vi "Administrator Console.vi"(8 "error in (no error)":errorcluster, 11 "Message Queues":T1) -> (0 "error out":errorcluster)   [LabVIEW 2024]
doc: "This VI is a user interface VI and is used to configure the server."
uses:
  Shared/Message Queue/Server Message Queues.ctl
  Shared/Message Queue/Message Cluster.ctl
  Controls/Server/Administrator Console - Data.ctl
  Shared/User Event - Stop.lvlib
  Shared/Message Queue.lvlib
panel:
  in  "Close":bool
  in  "Subsystems and I/O Points":string(tree)="..."
  in  "Configure Data Archiving":bool
  in  "Configure System":bool
  # "The Subsystem and I/O Points box lists every subsystem in the server and its I/O points. You can expand a subsystem to view its I/O points . Use the configuration buttons to modify the server."
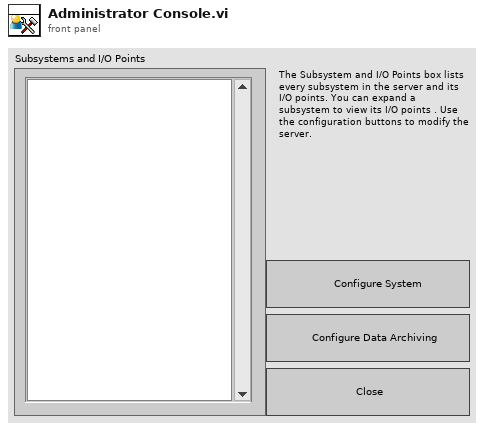
[diagram p1: front panel]
types:
  T1 = typedef "Message Queue.lvlib/Server Message Queues.ctl" = cluster{"UI":refnum<queue>, "Archive":refnum<queue>, "Shared Variable Management":refnum<queue>, "Administrator Console":refnum<queue>}
  T2 = typedef "Administrator Console - Data.ctl" = cluster{"Administrator Console Exit Handler":refnum<user-event>, "Server Message Queues":T1, "Subsystems Tree Control":refnum<vi>}
  T3 = typedef "Subsystem IO Attributes.ctl" = cluster{"Name":string, "Data Type":enum32{"u32BitField", "bool", "double", "string", "int8", "uint8", "int16", "uint16", "int32", "uint32", "int64", "uint64", "single", "double waveform", "int16 waveform", "array of boolean", "array of int8", "array of uint8", "array of int16", "array of uint16", "array of int32", "array of uint32", "array of int64", "array of uint64", "array of single", "array of double", "array of double waveform", "array of int16 waveform", "array of string", "variant", "timestamp", "fixed point", "custom"}, "Access Type":enum32{"Read only", "Write only", "Read/write"}, "Alarm Enabled?":bool, "Logging Enabled?":bool, "Logging Attributes":T4, "Alarm Attributes":T5}
  T4 = typedef "Subsystem IO Logging Attributes.ctl" = cluster{"log data? (F)":bool, "log alarms & events? (F)":bool}
  T5 = typedef "Subsystem IO Alarm Attributes.ctl" = cluster{"Hi:enable? (F)":bool, "Hi:name":string, "Hi:level/change":dbl, "Lo:enable? (F)":bool, "Lo:name":string, "Lo:level/change":dbl, "Boolean:enable? (F)":bool, "Boolean:name":string, "Boolean:value":bool, "BadStatus:enable? (F)":bool, "BadStatus:name":string}
  T6 = typedef "System Configuration.ctl" = cluster{"Name":string, "Description":string, "Logging Computer Name":string, "Logging Database Name":string, "Logging Database Path":path, "Archive Computer Name":string, "Archive Database Name":string, "Archive Database Path":path, "Lifespan (days)":u32, "Archive Enabled":bool, "Archive Interval (hours)":u32, "Subsystems":T7[]}
  T7 = typedef "Subsystem Configuration.ctl" = cluster{"Name":string, "Root URL":refnum<k21>}
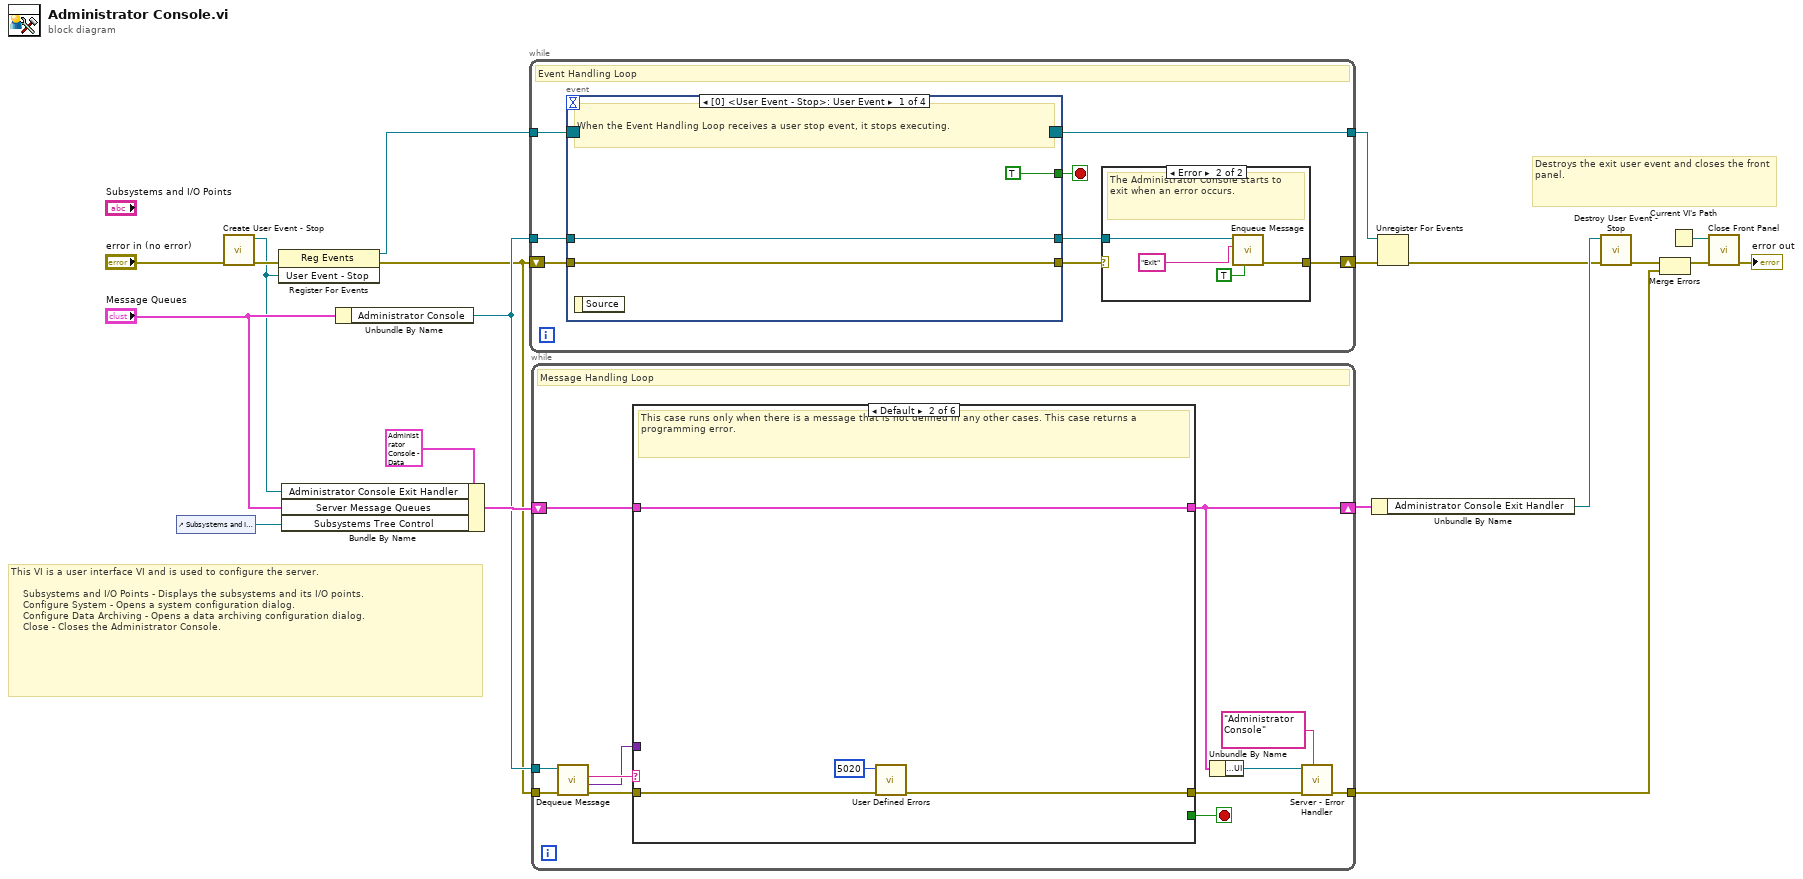
[diagram p0: block diagram]
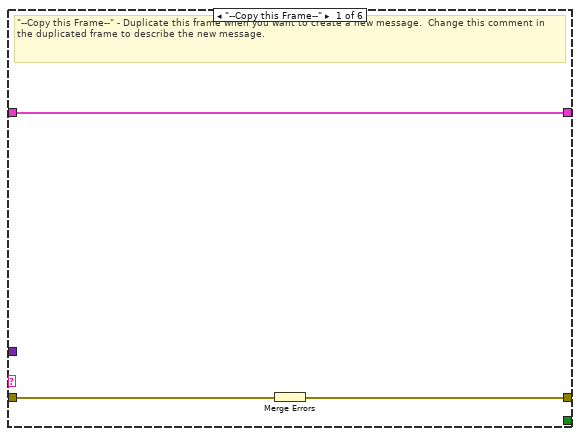
[diagram p2: hidden frame]
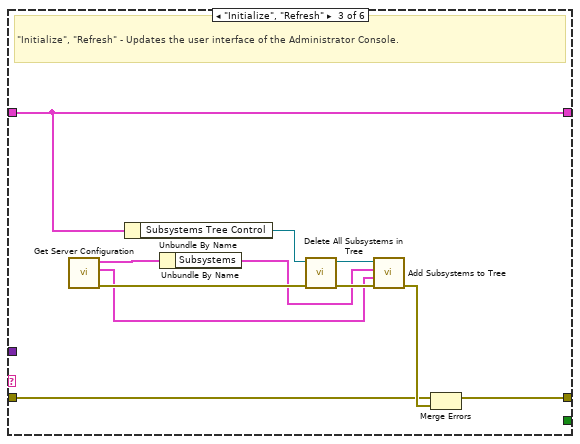
[diagram p3: hidden frame]
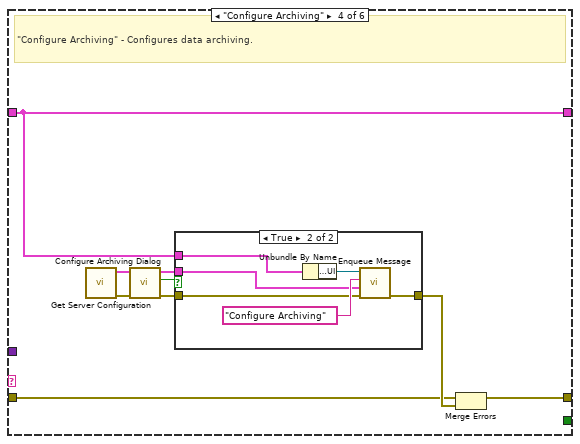
[diagram p4: hidden frame]
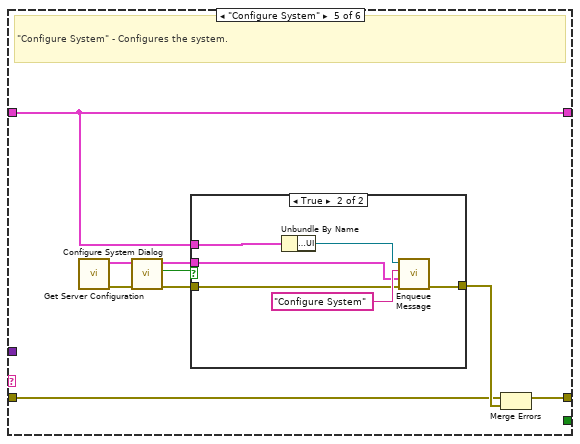
[diagram p6: hidden frame]
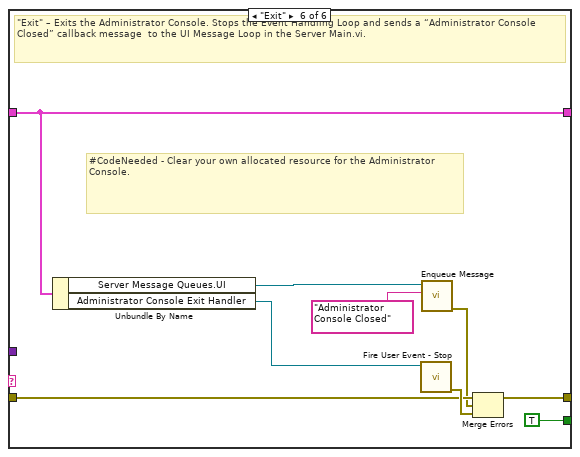
[diagram p8: hidden frame]
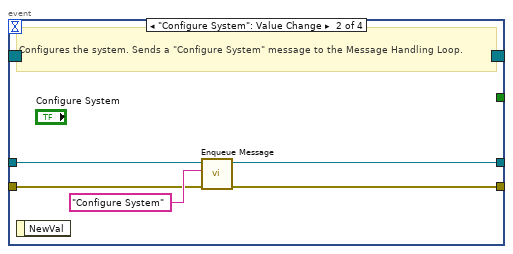
[diagram p10: hidden frame]
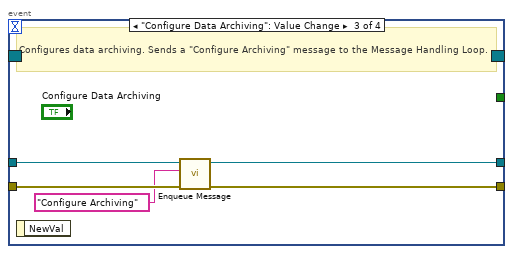
[diagram p11: hidden frame]
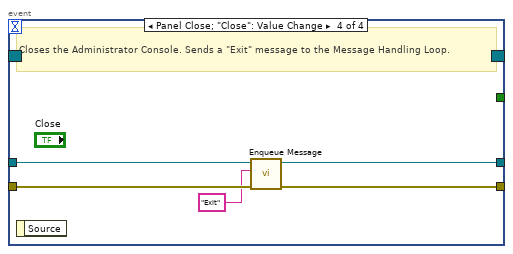
[diagram p12: hidden frame]
diagram:
  # "Destroys the exit user event and closes the front panel."
  # "This VI is a user interface VI and is used to configure the server.  \n\n    Subsystems and I/O Points - Displays the subsystems and its I/O points.\n    Configure System - Opens a system configuration dialog. \n    Configure Data Archiving - Opens a data archiving configuration dialog.\n    Close - Closes the Administrator Console."
  n1 = control-ref of="Subsystems and I/O Points"() -> (w12:refnum<vi>)
  n2 = call "Create User Event - Stop.vi"("error in (no error)"="error in (no error)") -> ("error out"=w4:errorcluster, "User Event - Stop"=w2:refnum<user-event>)  [unwired: 9 in]
  n3 = register-events(error in=w4, w2) -> (reference out=w1:refnum<event-registration>, error out=w3:errorcluster)  [unwired: 1 in]
  n4 = Bundle By Name(cluster=T2 {"Administrator Console Exit Handler"=refnum, "Server Message Queues"={"UI"=refnum, "Archive"=refnum, "Shared Variable Management"=refnum, "Administrator Console"=refnum}, "Subsystems Tree Control"=refnum} ("Administrator Console - Data"), "Administrator Console Exit Handler"=w2, "Server Message Queues"="Message Queues", "Subsystems Tree Control"=w12) -> (w20:T2)
  n5 = Unbundle By Name("Message Queues") -> ("Administrator Console"=w8:refnum<queue>)
  n6 = while {
    shift-right: [w22] -> w15
    shift-left: w3 -> [w27]
    tunnel: w8 -> [w26]
    tunnel: w1 -> [w25]
    tunnel: [w24] -> w14
    stop <- w28 stop-if-true
    # "Event Handling Loop"
    n7 = event shown="[0] <User Event - Stop>: User Event" {
      selector: w25 -> [_ _ _ _]
      dyn-events: [_ _ _ _] -> w24
      timeout: _ -> [_ _ _ _]
      tunnel: [TRUE _ _ _] -> w28
      tunnel: w27 -> [w35 w40 w46 w51]
      tunnel: [w35 w39 w43 w50] -> w23
      tunnel: w26 -> [w34 w38 w45 w49]
      tunnel: [w34 w37 w42 w48] -> w21
      event User Event {
        # "When the Event Handling Loop receives a user stop event, it stops executing."
        n8 = event-data() -> ()  [unwired: 1 in, 1 out]
      }
      event "Configure System": Value Change {
        # "Configures the system. Sends a \"Configure System\" message to the Message Handling Loop."
        n9 = event-data() -> ()  [unwired: 1 in, 1 out]
        n10 = call "Enqueue Message.vi"("error in (no error)"=w40, "Message"="Configure System", "Message Queue"=w38) -> ("error out"=w39:errorcluster, "dup Message Queue"=w37:refnum<queue>)  [unwired: 7 in]
      }
      event "Configure Data Archiving": Value Change {
        # "Configures data archiving. Sends a \"Configure Archiving\" message to the Message Handling Loop."
        n11 = event-data() -> ()  [unwired: 1 in, 1 out]
        n12 = call "Enqueue Message.vi"("error in (no error)"=w46, "Message"="Configure Archiving", "Message Queue"=w45) -> ("error out"=w43:errorcluster, "dup Message Queue"=w42:refnum<queue>)  [unwired: 7 in]
      }
      event Panel Close; "Close": Value Change {
        # "Closes the Administrator Console. Sends a \"Exit\" message to the Message Handling Loop."
        n13 = event-data() -> ()  [unwired: 1 in, 1 out]
        n14 = call "Enqueue Message.vi"("error in (no error)"=w51, "Message"="Exit", "Message Queue"=w49) -> ("error out"=w50:errorcluster, "dup Message Queue"=w48:refnum<queue>)  [unwired: 7 in]
      }
    }
    n15 = case "Event Handling Loop Error Handling" shown="Error" w23 {
      selector: w23 -> [w29 _]
      tunnel: w21 -> [_ w31]
      tunnel: [w29 w30] -> w22
      frame No Error {
        # "The Administrator Console does nothing when no error occurs."
      }
      frame Error {
        # "The Administrator Console starts to exit when an error occurs."
        n16 = call "Enqueue Message.vi"("Priority Message? (F)"=TRUE, "Message"="Exit", "Message Queue"=w31) -> ("error out"=w30:errorcluster)  [unwired: 7 in, 1 out]
      }
    }
  }
  n17 = while {
    shift-right: [w53] -> w19
    shift-left: w20 -> [w55]
    tunnel: w3 -> [w62]
    tunnel: [w57] -> w5
    tunnel: w8 -> [w52]
    stop <- w56 stop-if-true
    # "Message Handling Loop"
    n18 = call "Dequeue Message.vi"("error in (no error)"=w62, "Message Queue"=w52) -> ("error out"=w63:errorcluster, "Message Data"=w60:variant, "Message"=w61:string)  [unwired: 6 in, 1 out]
    n19 = case shown="Default" w61 {
      tunnel: w55 -> [w66 w70 w80 w83 w99 w122]
      tunnel: [w66 w70 w80 w83 w99 w122] -> w53
      tunnel: w63 -> [w65 w67 w72 w82 w98 w117]
      tunnel: w60 -> [_ _ _ _ _ _]
      tunnel: [w64 w68 w71 w90 w106 w120] -> w58
      tunnel: [_ _ _ _ _ TRUE] -> w56
      frame "--Copy this Frame--" {
        # "\"--Copy this Frame--\" - Duplicate this frame when you want to create a new message.  Change this comment in the duplicated frame to describe the new message."
        n20 = Merge Errors(w65) -> (w64:errorcluster)
      }
      frame Default {
        # "This case runs only when there is a message that is not defined in any other cases. This case returns a programming error."
        n21 = call "User Defined Errors.vi"("error in (no error)"=w67, "Error Code (0)"=5020 ("error code (0)")) -> ("error out"=w68:errorcluster)  [unwired: 9 in]
      }
      frame "Initialize", "Refresh" {
        # "\"Initialize\", \"Refresh\" - Updates the user interface of the Administrator Console."
        n22 = call "Get Server Configuration.vi"() -> ("error out"=w75:errorcluster, "Subsystem I/O Attributes"=w74:T3[], "System Configuration"=w76:T6)  [unwired: 9 in]
        n23 = Unbundle By Name(w80) -> ("Subsystems Tree Control"=w79:refnum<vi>)
        n24 = Unbundle By Name(w76) -> ("Subsystems"=w73:T7[])
        n25 = call "Delete All Subsystems in Tree.vi"("error in (no error)"=w75, "Tree Control"=w79) -> ("error out"=w77:errorcluster, "dup Tree Control"=w78:refnum<vi>)  [unwired: 8 in]
        n26 = call "Add Subsystems to Tree.vi"("error in (no error)"=w77, "Subsystem I/O Attributes"=w74, "Subsystems"=w73, "Tree Control"=w78) -> ("error out"=w81:errorcluster)  [unwired: 6 in, 1 out]
        n27 = Merge Errors(w72, w81) -> (w71:errorcluster)
      }
      frame "Configure Archiving" {
        # "\"Configure Archiving\" - Configures data archiving."
        n28 = call "Get Server Configuration.vi"() -> ("error out"=w84:errorcluster, "System Configuration"=w85:T6)  [unwired: 9 in, 1 out]
        n29 = call "Configure Archiving Dialog.vi"("error in (no error)"=w84, "System Configuration In"=w85) -> ("error out"=w88:errorcluster, "Changed?"=w87:bool, "System Configuration Out"=w86:T6)  [unwired: 7 in]
        n30 = case shown="True" w87 {
          tunnel: w88 -> [w91 w94]
          tunnel: w86 -> [_ w95]
          tunnel: [w91 w96] -> w89
          tunnel: w83 -> [_ w92]
          frame False {
          }
          frame True {
            n31 = Unbundle By Name(w92) -> ("Server Message Queues.UI"=w93:refnum<queue>)
            n32 = call "Enqueue Message.vi"("error in (no error)"=w94, "Message Data"=w95, "Message"="Configure Archiving", "Message Queue"=w93) -> ("error out"=w96:errorcluster)  [unwired: 6 in, 1 out]
          }
        }
        n33 = Merge Errors(w82, w89) -> (w90:errorcluster)
      }
      frame "Configure System" {
        # "\"Configure System\" - Configures the system."
        n34 = call "Get Server Configuration.vi"() -> ("error out"=w101:errorcluster, "System Configuration"=w100:T6)  [unwired: 9 in, 1 out]
        n35 = call "Configure System Dialog.vi"("error in (no error)"=w101, "System Configuration In"=w100) -> ("error out"=w104:errorcluster, "Changed?"=w103:bool, "System Configuration Out"=w102:T6)  [unwired: 5 in, 2 out]
        n36 = case shown="True" w103 {
          tunnel: w104 -> [w107 w111]
          tunnel: w102 -> [_ w112]
          tunnel: [w107 w110] -> w105
          tunnel: w99 -> [_ w108]
          frame False {
          }
          frame True {
            n37 = Unbundle By Name(w108) -> ("Server Message Queues.UI"=w109:refnum<queue>)
            n38 = call "Enqueue Message.vi"("error in (no error)"=w111, "Message Data"=w112, "Message"="Configure System", "Message Queue"=w109) -> ("error out"=w110:errorcluster)  [unwired: 6 in, 1 out]
          }
        }
        n39 = Merge Errors(w98, w105) -> (w106:errorcluster)
      }
      frame "Exit" {
        # "#CodeNeeded - Clear your own allocated resource for the Administrator Console."
        # "\"Exit\" – Exits the Administrator Console. Stops the Event Handling Loop and sends a “Administrator Console Closed” callback message  to the UI Message Loop in the Server Main.vi."
        n40 = Unbundle By Name(w122) -> ("Server Message Queues.UI"=w116:refnum<queue>, "Administrator Console Exit Handler"=w121:refnum<user-event>)
        n41 = call "Fire User Event - Stop.vi"("User Event - Stop"=w121) -> ("error out"=w119:errorcluster)  [unwired: 10 in]
        n42 = call "Enqueue Message.vi"("Message"="Administrator Console Closed", "Message Queue"=w116) -> ("error out"=w115:errorcluster)  [unwired: 8 in, 1 out]
        n43 = Merge Errors(w117, w115, w119) -> (w120:errorcluster)
      }
    }
    n44 = Unbundle By Name(w53) -> ("Server Message Queues.UI"=w54:refnum<queue>)
    n45 = call "Server - Error Handler.vi"("Component"="Administrator Console", "error in (no error)"=w58, "Message Queue"=w54) -> ("error out"=w57:errorcluster)  [unwired: 8 in]
  }
  n46 = Unbundle By Name(w19) -> ("Administrator Console Exit Handler"=w18:refnum<user-event>)
  n47 = Unregister For Events(event registration refnum=w14, error in=w15) -> (error out=w7:errorcluster)
  n48 = call "Destroy User Event - Stop.vi"("error in (no error)"=w7, "User Event - Stop"=w18) -> ("error out"=w10:errorcluster)  [unwired: 9 in]
  n49 = Merge Errors(w10, w5) -> (w6:errorcluster)
  n50 = Current VI's Path() -> (path=w11:path)
  n51 = call "Close Front Panel.vi"("error in (no error)"=w6, "VI File Path"=w11) -> ("error out"=→"error out":errorcluster)  [unwired: 9 in]
